vi "obj_LuaVIEW Task List.vi"(0 "method":T6, 5 "message":string, 7 "state object ref in":T1, 9 "script index":i32, 11 "task identifier":string) -> (4 "task info":T2 {"handle mask" format="%.0b"; "allow mask" format="%.0b"; "signal flags" format="%.0b"}, 6 "task info list":T2[](array[typedef]) {"handle mask" format="%.0b"; "allow mask" format="%.0b"; "signal flags" format="%.0b"}, 8 "state object ref out":T1, 10 "set/ongoing":bool, 14 "wakeup occurrence":refnum<k4>, 15 "script info":T5)   [LabVIEW 2012]
doc: "Lists LuaVIEW tasks and allows operations on tasks in the list. A particular task is specified through its identifier and manipulated through a reference to its state object. \nThis VI is only marginally part of the API: those methods that are in common use by function VIs can be deemed safe for use provided that typedefs are used so as to be forward compatible with extension of the method enum or typedef clusters (only use unbundle/bundle by name, and so on).\n\nBeware that when using this VI to send a request or message, the receiving task's request occurrence, as returned by this VI, must be set. This unfortunate inconvenience was made mandatory to avoid the superfluous context switches that can occur when occurrences are set from within a non-reentrant object."
uses:
  typedefs/t_LuaVIEW Task List Methods.ctl
  typedefs/clusters/LuaVIEW Task Info.ctl
  typedefs/t_LuaVIEW Task Modes.ctl
  typedefs/t_LuaVIEW Reference.ctl
  typedefs/t_LuaVIEW Task State Pane.ctl
  typedefs/clusters/LuaVIEW Script Info.ctl
  typedefs/t_LuaVIEW Task State Methods.ctl
  typedefs/t_LuaVIEW Task Signals.ctl
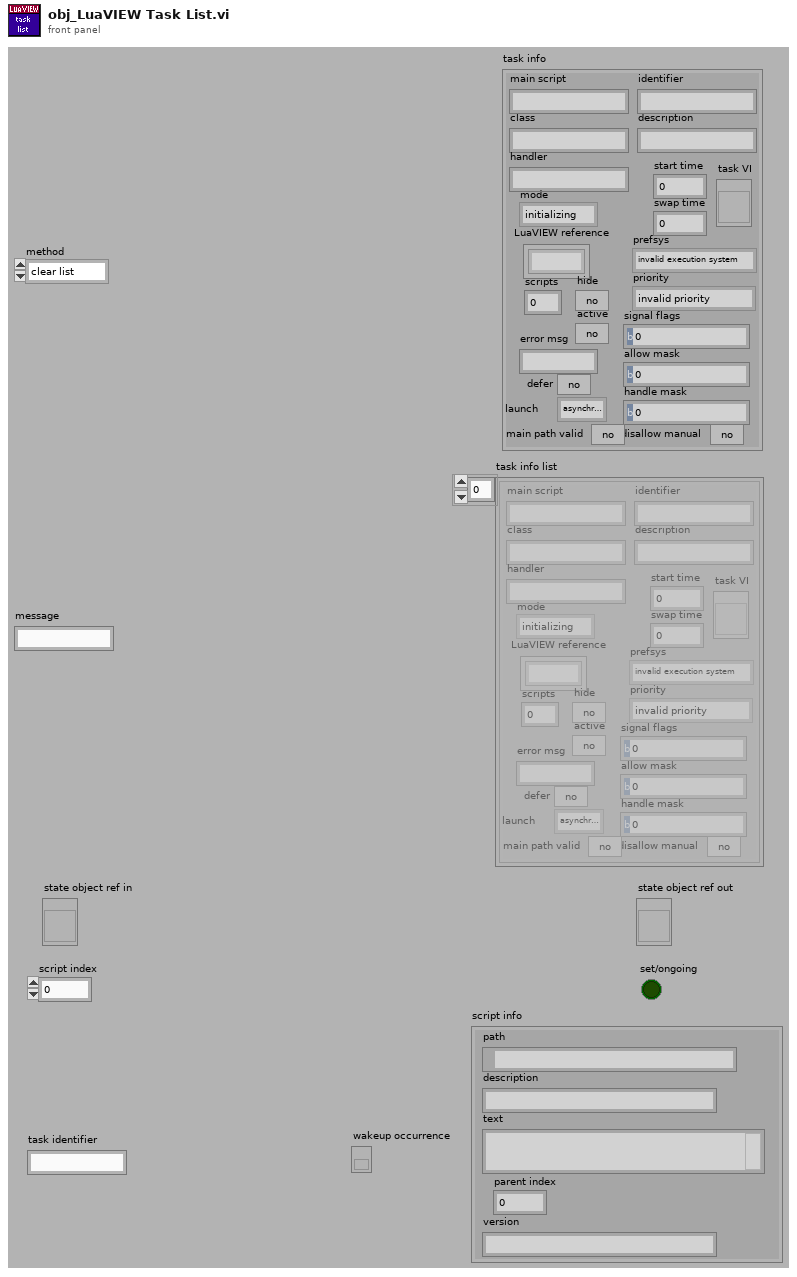
[diagram p1: front panel]
types:
  T1 = typedef "t_LuaVIEW Task State Pane.ctl" = refnum<vi>
  T2 = typedef "LuaVIEW Task Info.ctl" = cluster{"main script":string, "identifier":string, "class":string, "description":string, "mode":T3, "handler":string, "LuaVIEW reference":T4, "scripts":i32, "hide":bool, "active":bool, "error msg":string, "defer":bool, "launch":enum16{"asynchronous", "manual", "synchronous"}, "main path valid":bool, "start time":dbl, "swap time":dbl, "task VI":refnum<vi>, "prefsys":enum32{"invalid execution system", "user interface", "standard", "instrument i/o", "data acquisition", "other 1", "other 2", "same as caller"}, "priority":enum32{"invalid priority", "background priority", "normal priority", "above normal priority", "high priority", "time critical priority", "subroutine"}, "signal flags":u32, "allow mask":u32, "handle mask":u32, "disallow manual":bool}
  T3 = typedef "t_LuaVIEW Task Modes.ctl" = enum16{"initializing", "running", "executing", "paused", "error", "swapping"}
  T4 = typedef "t_LuaVIEW Reference.ctl" = refnum<k1>
  T5 = typedef "LuaVIEW Script Info.ctl" = cluster{"path":path, "description":string, "text":string, "parent index":i32, "version":string}
  T6 = typedef "t_LuaVIEW Task List Methods.ctl" = enum16{"clear list", "add", "test", "remove", "get ref", "get task info", "get list", "get script info", "ongoing?", "resume", "pause", "stop", "confirm", "message"}
  T7 = typedef "t_LuaVIEW Task State Methods.ctl" = enum16{"cleanup", "set initial", "set mode", "set active mode", "set error", "get task info", "get script info", "set signal", "clear signal", "test handled", "test delegated", "test signal", "handle signal", "delegate signal", "allow signal", "disallow signal", "disallow all", "signals?", "delegated signals?", "protection++", "protection--", "protection=0", "message", "next message", "pop message", "message available?", "force stop", "set swap preps", "apply swap preps"}
  T8 = typedef "t_LuaVIEW Task Signals.ctl" = enum32{"resume", "pause", "swap", "stop", "confirm"}
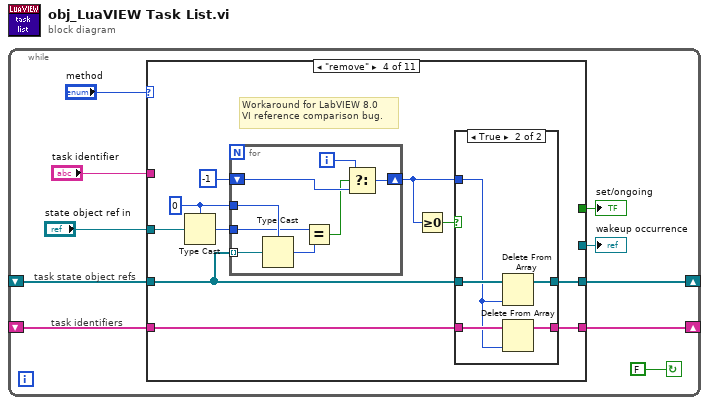
[diagram p0: block diagram]
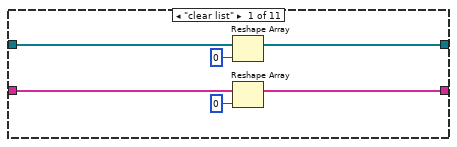
[diagram p2: hidden frame]
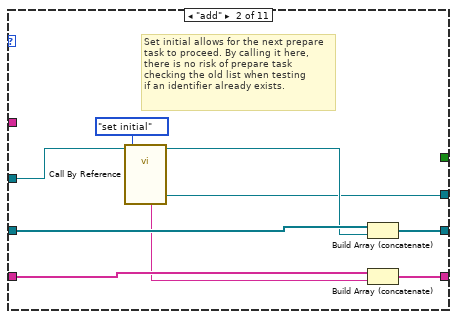
[diagram p3: hidden frame]
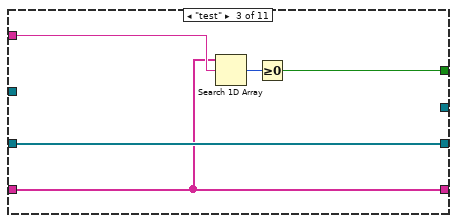
[diagram p4: hidden frame]
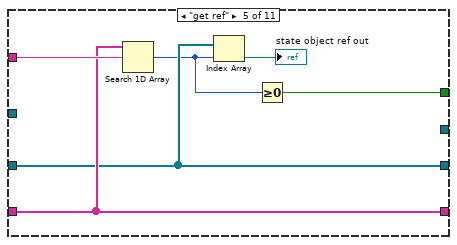
[diagram p6: hidden frame]
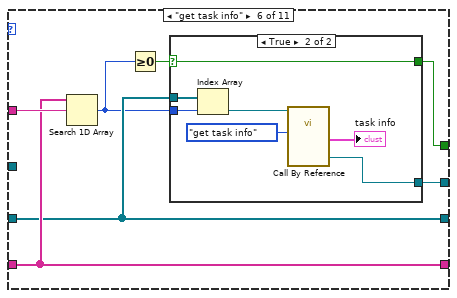
[diagram p7: hidden frame]
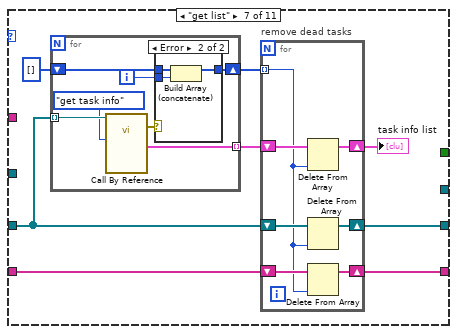
[diagram p9: hidden frame]
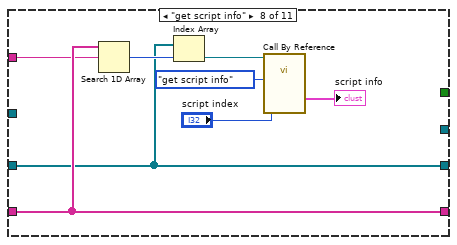
[diagram p11: hidden frame]
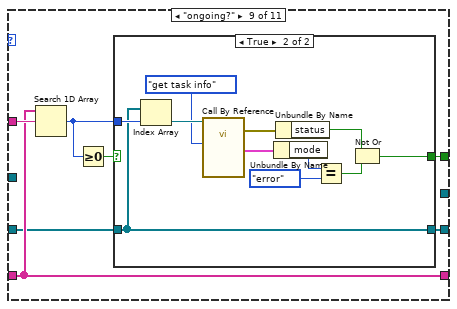
[diagram p12: hidden frame]
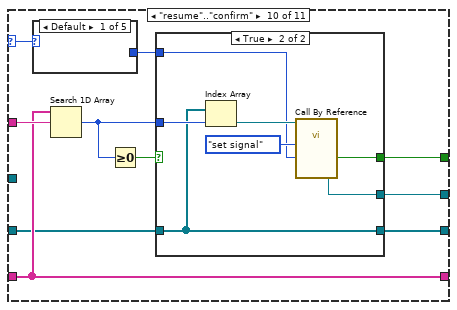
[diagram p14: hidden frame]
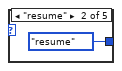
[diagram p15: hidden frame]
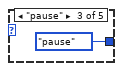
[diagram p16: hidden frame]
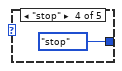
[diagram p17: hidden frame]
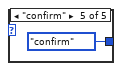
[diagram p18: hidden frame]
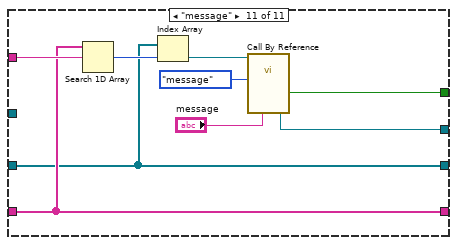
[diagram p20: hidden frame]
diagram:
  n1 = while {
    shift-right: [w1] -> _
    shift-left: _ -> [w8]
    shift-right: [w6] -> _
    shift-left: _ -> [w7]
    stop <- FALSE continue-if-true
    # "task identifiers"
    # "task state object refs"
    n2 = case shown="\"remove\"" "method" {
      selector: "method" -> [_ _ _ _ _ _ _ _ _ w132 _]
      tunnel: w8 -> [w12 w24 w28 w33 w59 w66 w80 w108 w113 w138 w159]
      tunnel: [w15 w25 w28 w40 w59 w66 w78 w108 w111 w135 w159] -> w1
      tunnel: w7 -> [w13 w19 w27 w37 w60 w67 w81 w110 w116 w139 w161]
      tunnel: [w11 w23 w27 w39 w60 w67 w79 w110 w116 w139 w161] -> w6
      tunnel: "task identifier" -> [_ _ w30 _ w61 w68 _ w103 w117 w140 w162]
      tunnel: [_ _ w26 _ w57 w62 _ _ w114 w137 w156] -> w4
      tunnel: [_ w18 _ _ _ w65 _ _ _ w136 w154] -> w3
      tunnel: "state object ref in" -> [_ w21 _ w34 _ _ _ _ _ _ _]
      frame "clear list" {
        n3 = Reshape Array(w12, 0 ("dimension size")) -> (w15:T1[])
        n4 = Reshape Array(w13, 0 ("dimension size")) -> (w11:string[])
      }
      frame "add" {
        # "Set initial allows for the next prepare\ntask to proceed. By calling it here,\nthere is no risk of prepare task\nchecking the old list when testing\nif an identifier already exists."
        n5 = call-by-ref "?"(reference=w21, "method"=t_LuaVIEW_Task_State_Methods."set initial" ("method (get)")) -> (reference out=w20:T1, "string out"=w17:string, "wakeup occurrence"=w18:refnum<k4>)  [unwired: 11 in, 4 out]
        n6 = Build Array (concatenate)(w24, w20) -> (w25:T1[])
        n7 = Build Array (concatenate)(w19, w17) -> (w23:string[])
      }
      frame "test" {
        n8 = Search 1D Array(1D array=w27, element=w30) -> (index of element=w29:i32)  [unwired: 1 in]
        n9 = Greater Or Equal To 0?(x=w29) -> (x >= 0?=w26:bool)
      }
      frame "remove" {
        w32 = u32 0
        # "Workaround for LabVIEW 8.0\nVI reference comparison bug."
        n10 = Type Cast(type=w32, x=w34) -> (*(type *) &x=w31:u32)
        n11 = for {
          shift-right: [w42] -> w35
          shift-left: -1 -> [w44]
          tunnel: w33 -> [w48] mode=indexing
          tunnel: w32 -> [w47]
          tunnel: w31 -> [w46]
          i -> [w43]
          n12 = Type Cast(type=w47, x=w48) -> (*(type *) &x=w45:u32)
          n13 = Equal?(x=w46, y=w45) -> (x = y?=w41:bool)
          n14 = Select(t=w43, s=w41, f=w44) -> (s? t:f=w42:i32)
        }
        n15 = Greater Or Equal To 0?(x=w35) -> (x >= 0?=w38:bool)
        n16 = case shown="True" w38 {
          tunnel: [w50 w55] -> w40
          tunnel: w37 -> [w49 w54]
          tunnel: [w49 w53] -> w39
          tunnel: w35 -> [_ w51]
          tunnel: w33 -> [w50 w52]
          frame False {
          }
          frame True {
            n17 = Delete From Array(array=w52, index=w51) -> (array with subset deleted=w55:T1[])  [unwired: 1 in, 1 out]
            n18 = Delete From Array(array=w54, index=w51) -> (array with subset deleted=w53:string[])  [unwired: 1 in, 1 out]
          }
        }
      }
      frame "get ref" {
        n19 = Search 1D Array(1D array=w60, element=w61) -> (index of element=w56:i32)  [unwired: 1 in]
        n20 = Index Array(array=w59, index=w56) -> (element=→"state object ref out":T1)
        n21 = Greater Or Equal To 0?(x=w56) -> (x >= 0?=w57:bool)
      }
      frame "get task info" {
        n22 = Search 1D Array(1D array=w67, element=w68) -> (index of element=w64:i32)  [unwired: 1 in]
        n23 = Greater Or Equal To 0?(x=w64) -> (x >= 0?=w63:bool)
        n24 = case shown="True" w63 {
          selector: w63 -> [w69 w72]
          tunnel: w66 -> [_ w76]
          tunnel: [_ w74] -> w65
          tunnel: w64 -> [_ w73]
          tunnel: [w69 w72] -> w62
          frame False {
          }
          frame True {
            n25 = Index Array(array=w76, index=w73) -> (element=w71:T1)
            n26 = call-by-ref "?"(reference=w71, "method"=t_LuaVIEW_Task_State_Methods."get task info") -> ("task info {get task info}"=→"task info":T2, "wakeup occurrence"=w74:refnum<k4>)  [unwired: 11 in, 5 out]
          }
        }
      }
      frame "get list" {
        n27 = for {
          tunnel: w80 -> [w97] mode=indexing
          tunnel: [w98] -> w82 mode=indexing
          shift-right: [w93] -> w83
          shift-left: i32[] [] -> [w94]
          i -> [w92]
          n28 = call-by-ref "?"(reference=w97, "method"=t_LuaVIEW_Task_State_Methods."get task info") -> (error out=w95:errorcluster, "task info {get task info}"=w98:T2)  [unwired: 11 in, 5 out]
          n29 = case shown="Error" w95 {
            tunnel: w94 -> [w99 w102]
            tunnel: [w99 w101] -> w93
            tunnel: w92 -> [_ w100]
            frame No Error {
            }
            frame Error {
              n30 = Build Array (concatenate)(w102, w100) -> (w101:i32[])
            }
          }
        }
        n31 = for "remove dead tasks" {
          tunnel: w83 -> [w85] mode=indexing
          shift-right: [w90] -> w77
          shift-left: w82 -> [w91]
          shift-right: [w86] -> w79
          shift-left: w81 -> [w87]
          shift-right: [w88] -> w78
          shift-left: w80 -> [w89]
          n32 = Delete From Array(array=w91, index=w85) -> (array with subset deleted=w90:T2[])  [unwired: 1 in, 1 out]
          n33 = Delete From Array(array=w89, index=w85) -> (array with subset deleted=w88:T1[])  [unwired: 1 in, 1 out]
          n34 = Delete From Array(array=w87, index=w85) -> (array with subset deleted=w86:string[])  [unwired: 1 in, 1 out]
        }
        "task info list" <- w77
      }
      frame "get script info" {
        n35 = Search 1D Array(1D array=w110, element=w103) -> (index of element=w109:i32)  [unwired: 1 in]
        n36 = Index Array(array=w108, index=w109) -> (element=w105:T1)
        n37 = call-by-ref "?"(reference=w105, "method"=t_LuaVIEW_Task_State_Methods."get script info", "script index"="script index") -> ("script info"=→"script info":T5)  [unwired: 10 in, 6 out]
      }
      frame "ongoing?" {
        n38 = Search 1D Array(1D array=w116, element=w117) -> (index of element=w112:i32)  [unwired: 1 in]
        n39 = Greater Or Equal To 0?(x=w112) -> (x >= 0?=w115:bool)
        n40 = case shown="True" w115 {
          selector: w115 -> [w119 _]
          tunnel: [w119 w122] -> w114
          tunnel: w113 -> [w118 w124]
          tunnel: [w118 w124] -> w111
          tunnel: w112 -> [_ w130]
          frame False {
          }
          frame True {
            n41 = Index Array(array=w124, index=w130) -> (element=w129:T1)
            n42 = call-by-ref "?"(reference=w129, "method"=t_LuaVIEW_Task_State_Methods."get task info") -> (error out=w125:errorcluster, "task info {get task info}"=w127:T2)  [unwired: 11 in, 5 out]
            n43 = Unbundle By Name(w127) -> ("mode"=w123:T3)
            n44 = Unbundle By Name(w125) -> ("status"=w121:bool)
            n45 = Equal?(x=w123, y=t_LuaVIEW_Task_Modes."error" ("mode")) -> (x = y?=w120:bool)
            n46 = Not Or(1:w120, 2:w121) -> (0:w122:bool)
          }
        }
      }
      frame "resume".."confirm" {
        n47 = case shown="Default" w132 {
          tunnel: [_ t_LuaVIEW_Task_Signals."resume" t_LuaVIEW_Task_Signals."pause" t_LuaVIEW_Task_Signals."stop" t_LuaVIEW_Task_Signals."confirm"] -> w131
          frame Default {
          }
          frame "resume" {
          }
          frame "pause" {
          }
          frame "stop" {
          }
          frame "confirm" {
          }
        }
        n48 = Search 1D Array(1D array=w139, element=w140) -> (index of element=w134:i32)  [unwired: 1 in]
        n49 = Greater Or Equal To 0?(x=w134) -> (x >= 0?=w133:bool)
        n50 = case shown="True" w133 {
          selector: w133 -> [w145 _]
          tunnel: w134 -> [_ w153]
          tunnel: w138 -> [w146 w148]
          tunnel: [w145 w150] -> w137
          tunnel: [_ w149] -> w136
          tunnel: [w146 w148] -> w135
          tunnel: w131 -> [_ w147]
          frame False {
          }
          frame True {
            n51 = Index Array(array=w148, index=w153) -> (element=w152:T1)
            n52 = call-by-ref "?"(reference=w152, "method"=t_LuaVIEW_Task_State_Methods."set signal", "signal"=w147) -> ("set/available/pending"=w150:bool, "wakeup occurrence"=w149:refnum<k4>)  [unwired: 10 in, 5 out]
          }
        }
      }
      frame "message" {
        n53 = Search 1D Array(1D array=w161, element=w162) -> (index of element=w160:i32)  [unwired: 1 in]
        n54 = Index Array(array=w159, index=w160) -> (element=w158:T1)
        n55 = call-by-ref "?"(reference=w158, "method"=t_LuaVIEW_Task_State_Methods."message", "string in"="message") -> ("set/available/pending"=w156:bool, "wakeup occurrence"=w154:refnum<k4>)  [unwired: 10 in, 5 out]
      }
    }
    "set/ongoing" <- w4
    "wakeup occurrence" <- w3
  }
